vi "CAN_Get_Ref.vi"(8 "error in (no error)":errorcluster) -> (0 "error out":errorcluster, 3 "CAN_Jaguars_ref":T2)   [LabVIEW 2009, in "OWNCAN.lvlib"]
uses:
  OWNCAN.lvlib
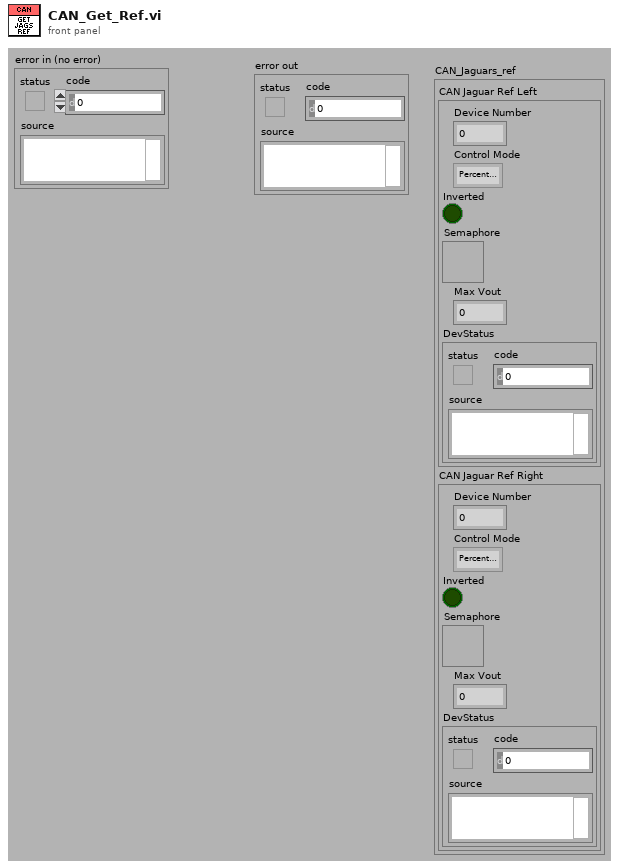
[diagram p1: front panel]
types:
  T1 = typedef "Semaphore RefNum" = refnum<k1>
  T2 = cluster{"CAN Jaguar Ref Left":cluster{"Device Number":u8, "Control Mode":enum16{"Percent VBus", "Speed", "Position", "Current"}, "Inverted":bool, "Semaphore":T1, "Max Vout":dbl, "DevStatus":errorcluster}, "CAN Jaguar Ref Right":cluster{"Device Number":u8, "Control Mode":enum16{"Percent VBus", "Speed", "Position", "Current"}, "Inverted":bool, "Semaphore":T1, "Max Vout":dbl, "DevStatus":errorcluster}}
  T3 = cluster{"CAN Jaguar Ref Left":cluster{"Device Number":u8, "Control Mode":enum16{"Percent VBus", "Speed", "Position", "Current"}, "Inverted":bool, "Semaphore":refnum<k1>, "Max Vout":dbl, "DevStatus":errorcluster}, "CAN Jaguar Ref Right":cluster{"Device Number":u8, "Control Mode":enum16{"Percent VBus", "Speed", "Position", "Current"}, "Inverted":bool, "Semaphore":refnum<k1>, "Max Vout":dbl, "DevStatus":errorcluster}}
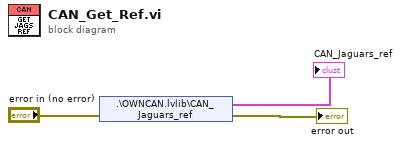
[diagram p0: block diagram]
diagram:
  n1 = shared-variable ".\\OWNCAN.lvlib\\CAN_Jaguars_ref"(error in="error in (no error)") -> (→"CAN_Jaguars_ref":T3, error out=→"error out":errorcluster)
